vi "_Destroy.vi"(8 "error in (no error)":errorcluster, 11 "Spectrometer iHR320 in":refnum<class "Spectrometer iHR320.lvclass">) -> (0 "error out":errorcluster)   [LabVIEW 2009, in "Spectrometer iHR320.lvclass"]
doc: "Superclass destructor: close all handles to and release all resources associated with this Instrument, then deallocate it. \n\nIMPORTANT: when destroying a class that inherits from Instrument, destroy your subclass first, and call the parent Instrument::_Destroy.vi LAST. This ensures your subclass destructor operates on a valid Instrument while it releases its resources."
uses:
  Spectrometer iHR320.lvclass
  Utility Classes/Scannable/Scannable.lvclass
  Spectrometer iHR320.lvclass/Spectrometer iHR320.ctl
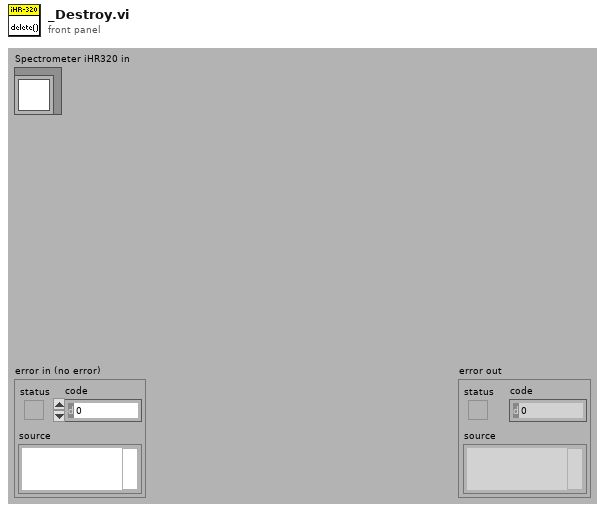
[diagram p1: front panel]
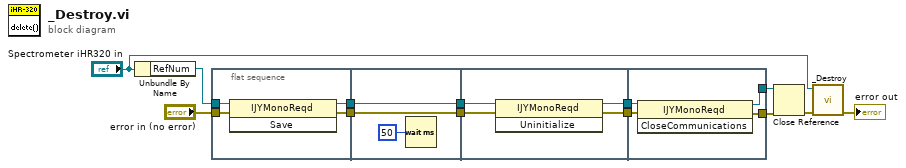
[diagram p0: block diagram]
diagram:
  n1 = Unbundle By Name("Spectrometer iHR320 in") -> ("RefNum"=w10:refnum<k7>)
  n2 = flat-sequence {
    tunnel: w10 -> [w17]
    tunnel: "error in (no error)" -> [w16]
    tunnel: [w15] -> w8
    tunnel: [w14] -> w7
    tunnel: w8 -> [w20]
    tunnel: w7 -> [w19]
    tunnel: [w20] -> w2
    tunnel: [w19] -> w1
    tunnel: [w24] -> w4
    tunnel: [w23] -> w3
    tunnel: w2 -> [w22]
    tunnel: w1 -> [w21]
    tunnel: [w28] -> w6
    tunnel: [w27] -> w5
    tunnel: w4 -> [w26]
    tunnel: w3 -> [w25]
    frame #0 {
      n3 = invoke class="IJYMonoReqd" method="Save"(reference=w17, error in=w16) -> (reference out=w14:refnum<k7>, error out=w15:errorcluster)  [unwired: 1 in, 1 out]
    }
    frame #1 {
      n4 = Wait (ms)(milliseconds to wait=u32 50) -> ()  [unwired: 1 out]
    }
    frame #2 {
      n5 = invoke class="IJYMonoReqd" method="Uninitialize"(reference=w21, error in=w22) -> (reference out=w23:refnum<k7>, error out=w24:errorcluster)  [unwired: 1 in, 1 out]
    }
    frame #3 {
      n6 = invoke class="IJYMonoReqd" method="CloseCommunications"(reference=w25, error in=w26) -> (reference out=w27:refnum<k7>, error out=w28:errorcluster)  [unwired: 1 in, 1 out]
    }
  }
  n7 = Close Reference(reference=w5, error in (no error)=w6) -> (error out=w12:errorcluster)
  n8 = call-parent "_Destroy.vi"("error in (no error)"=w12, "Instrument in"="Spectrometer iHR320 in") -> ("error out"=→"error out":errorcluster)  [unwired: 9 in]
